vi "Extract Label.vi"(11 "Statement in":string) -> (2 "Label":string, 3 "Statement out":string)   [LabVIEW 2017]
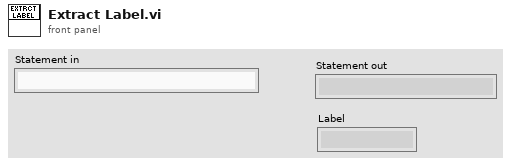
[diagram p1: front panel]
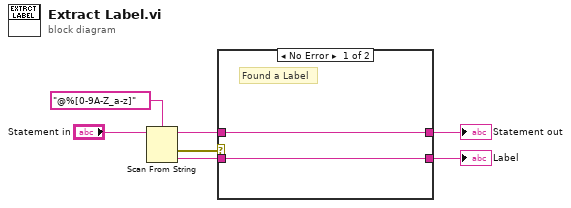
[diagram p0: block diagram]
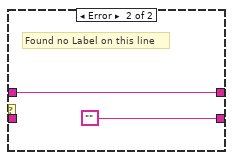
[diagram p2: hidden frame]
diagram:
  n1 = Scan From String(format string="@%[0-9A-Z_a-z]", input string="Statement in") -> (remaining string=w3:string, error out=w5:errorcluster, output 1=w4:string)  [unwired: 3 in, 1 out]
  n2 = case shown="No Error" w5 {
    tunnel: w4 -> [w8 _]
    tunnel: w3 -> [w9 w10]
    tunnel: [w9 w10] -> w2
    tunnel: [w8 ""] -> w1
    frame No Error {
      # "Found a Label"
    }
    frame Error {
      # "Found no Label on this line"
    }
  }
  "Statement out" <- w2
  "Label" <- w1
